vi "Initialize.vi"(8 "error in (no error)":errorcluster, 11 "User Interface in":refnum<class "User Interface.lvclass">) -> (0 "error out":errorcluster, 3 "User Interface out":refnum<class "User Interface.lvclass">)   [LabVIEW 2017, in "DSF Core.lvlib" / "User Interface.lvclass"]
uses:
  User Interface.lvclass
  User Interface.lvclass/User Interface.ctl
  User Interface Events/User Interface Events.lvclass
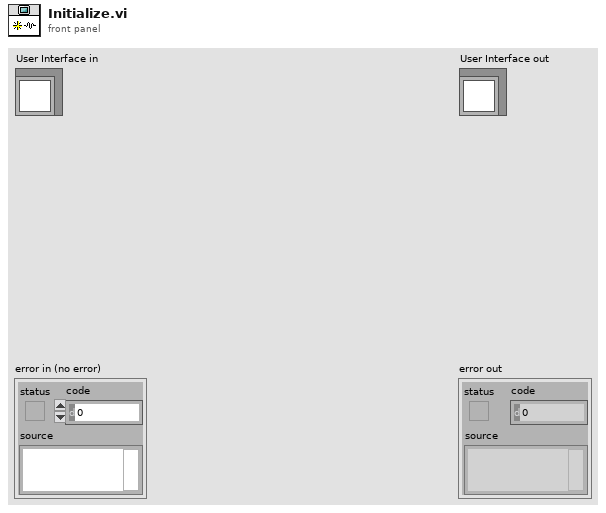
[diagram p1: front panel]
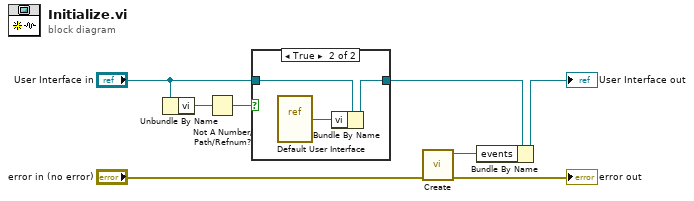
[diagram p0: block diagram]
diagram:
  n1 = Unbundle By Name("User Interface in") -> ("vi"=w8:refnum<vi>)
  n2 = Not A Number/Path/Refnum?(number/path/refnum=w8) -> (NaN/Path/Refnum?=w2:bool)
  n3 = case shown="True" w2 {
    tunnel: "User Interface in" -> [w9 w12]
    tunnel: [w9 w11] -> w3
    frame False {
    }
    frame True {
      n4 = vi-ref "Default User Interface.vi"() -> (w10:refnum<vi>)
      n5 = Bundle By Name(cluster=w12, "vi"=w10) -> (w11:refnum<class "User Interface.lvclass">)
    }
  }
  n6 = call "Create.vi"("error in (no error)"="error in (no error)") -> ("error out"=→"error out":errorcluster, "User Interface Events out"=w6:refnum<class "User Interface Events.lvclass">)  [unwired: 9 in]
  n7 = Bundle By Name(cluster=w3, "events"=w6) -> (→"User Interface out":refnum<class "User Interface.lvclass">)
